vi "Main_GEA3.vi"() -> ()   [LabVIEW 2021]
uses:
  Controles/Multiple_Read_ERD.ctl
  Controles/Read_ERD.ctl
  Controles/Write_Multiple_ERD.ctl
  Controles/Write_ERD.ctl
  Controles/Send_Message.ctl
  Controles/ERD_List.ctl
  Controles/Main_Machine_State.ctl
  Controles/ERD_Data_Boundled.ctl
  Controles/Command(ERD Loop Control).ctl
panel:
  in  "Pause(ms)":u32=100
  out "Rate":u32=100
  in  "Tab Control":enum32{"GEA3", "JSON", "Send Msg", "ERD List"}(tab)
  in  "Write ERD":T1 {"ERD" format="%x"}
  in  "Read ERD":i64[](array[numeric]) format="%x"
  in  "Read":bool
  in  "Write":bool caption="Read"
  in  "dst":i64=192 format="%x"
  out "Multiple_Result":T3 {"ERD Number" format="%x"}
  out "Version":T5
  in  "Json File Path":path
  out "Json":T4[](array[typedef]) {"ERD Number" format="%x"}
  in  "Send":bool caption="Read"
  in  "Send Message":T6={"dst"=192, "Command"=221, "Message"=""} {"Command" format="%x"; "dst" format="%x"}
  out "Message":string
  in  "ERD Default List":T7=[{"Boolean"=TRUE, "ERD Number"=2, "ERD Nanme"="Erd_UnitSerialNumber"}] {"ERD Number" format="%x"}
  in  "ERD's List Ticket Testing":T7=[{"Boolean"=TRUE, "ERD Number"=61497, "ERD Nanme"="Erd_UI_MachineStateEnter"}, {"Boolean"=TRUE, "ERD Number"=61498, "ERD Nanme"="Erd_UI_MachineStateExit"}, {"Boolean"=TRUE, "ERD Number"=61499, "ERD Nanme"="Erd_UI_CycleSelection"}] {"ERD Number" format="%x"}
  in  "Stop Button":bool
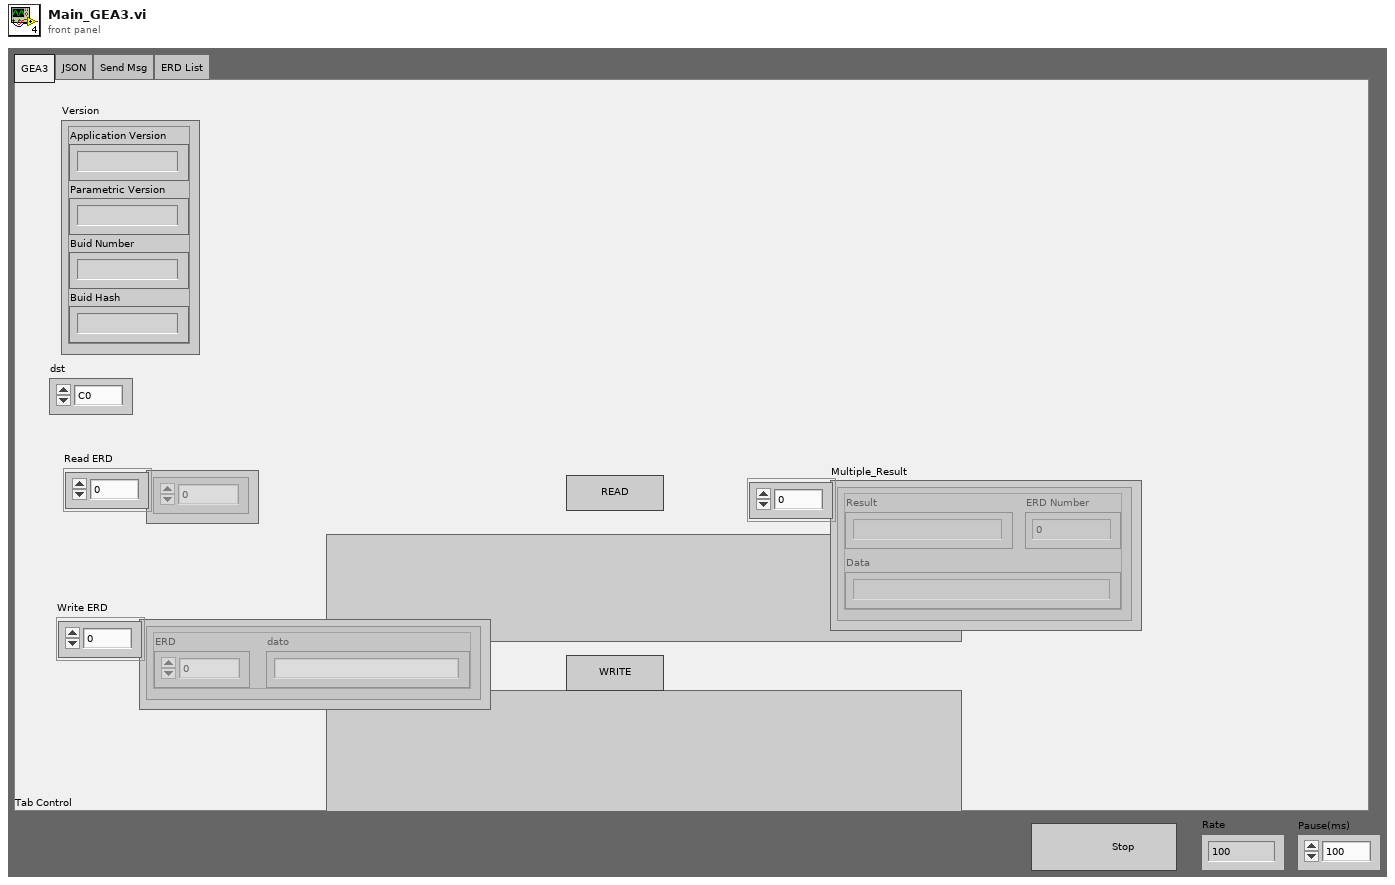
[diagram p1: front panel]
types:
  T1 = typedef "Write_Multiple_ERD.ctl" = T2[]
  T2 = typedef "Write_ERD.ctl" = cluster{"ERD":i64, "dato":string}
  T3 = typedef "Multiple_Read_ERD.ctl" = T4[]
  T4 = typedef "Read_ERD.ctl" = cluster{"Result":string, "ERD Number":i64, "Data":string}
  T5 = cluster{"Application Version":string, "Parametric Version":string, "Buid Number":string, "Buid Hash":string}
  T6 = typedef "Send_Message.ctl" = cluster{"dst":i64, "Command":i64, "Message":string}
  T7 = typedef "ERD_List.ctl" = cluster{"Boolean":bool, "ERD Number":i32, "ERD Nanme":string}[]
  T8 = typedef "ERD_Data_Boundled.ctl" = cluster{"Version":cluster{"Application Version":string, "Parametric Version":string, "Buid Number":string, "Buid Hash":string}}
  T9 = typedef "Main_Machine_State.ctl" = enum16{"Init", "Get Version", "Build ERD Read List", "Update UI", "Read ERDs", "Log Data", "Pause", "Shutdown"}
  T10 = typedef "Command(ERD Loop Control).ctl" = enum16{"Initialize", "Shutdown"}
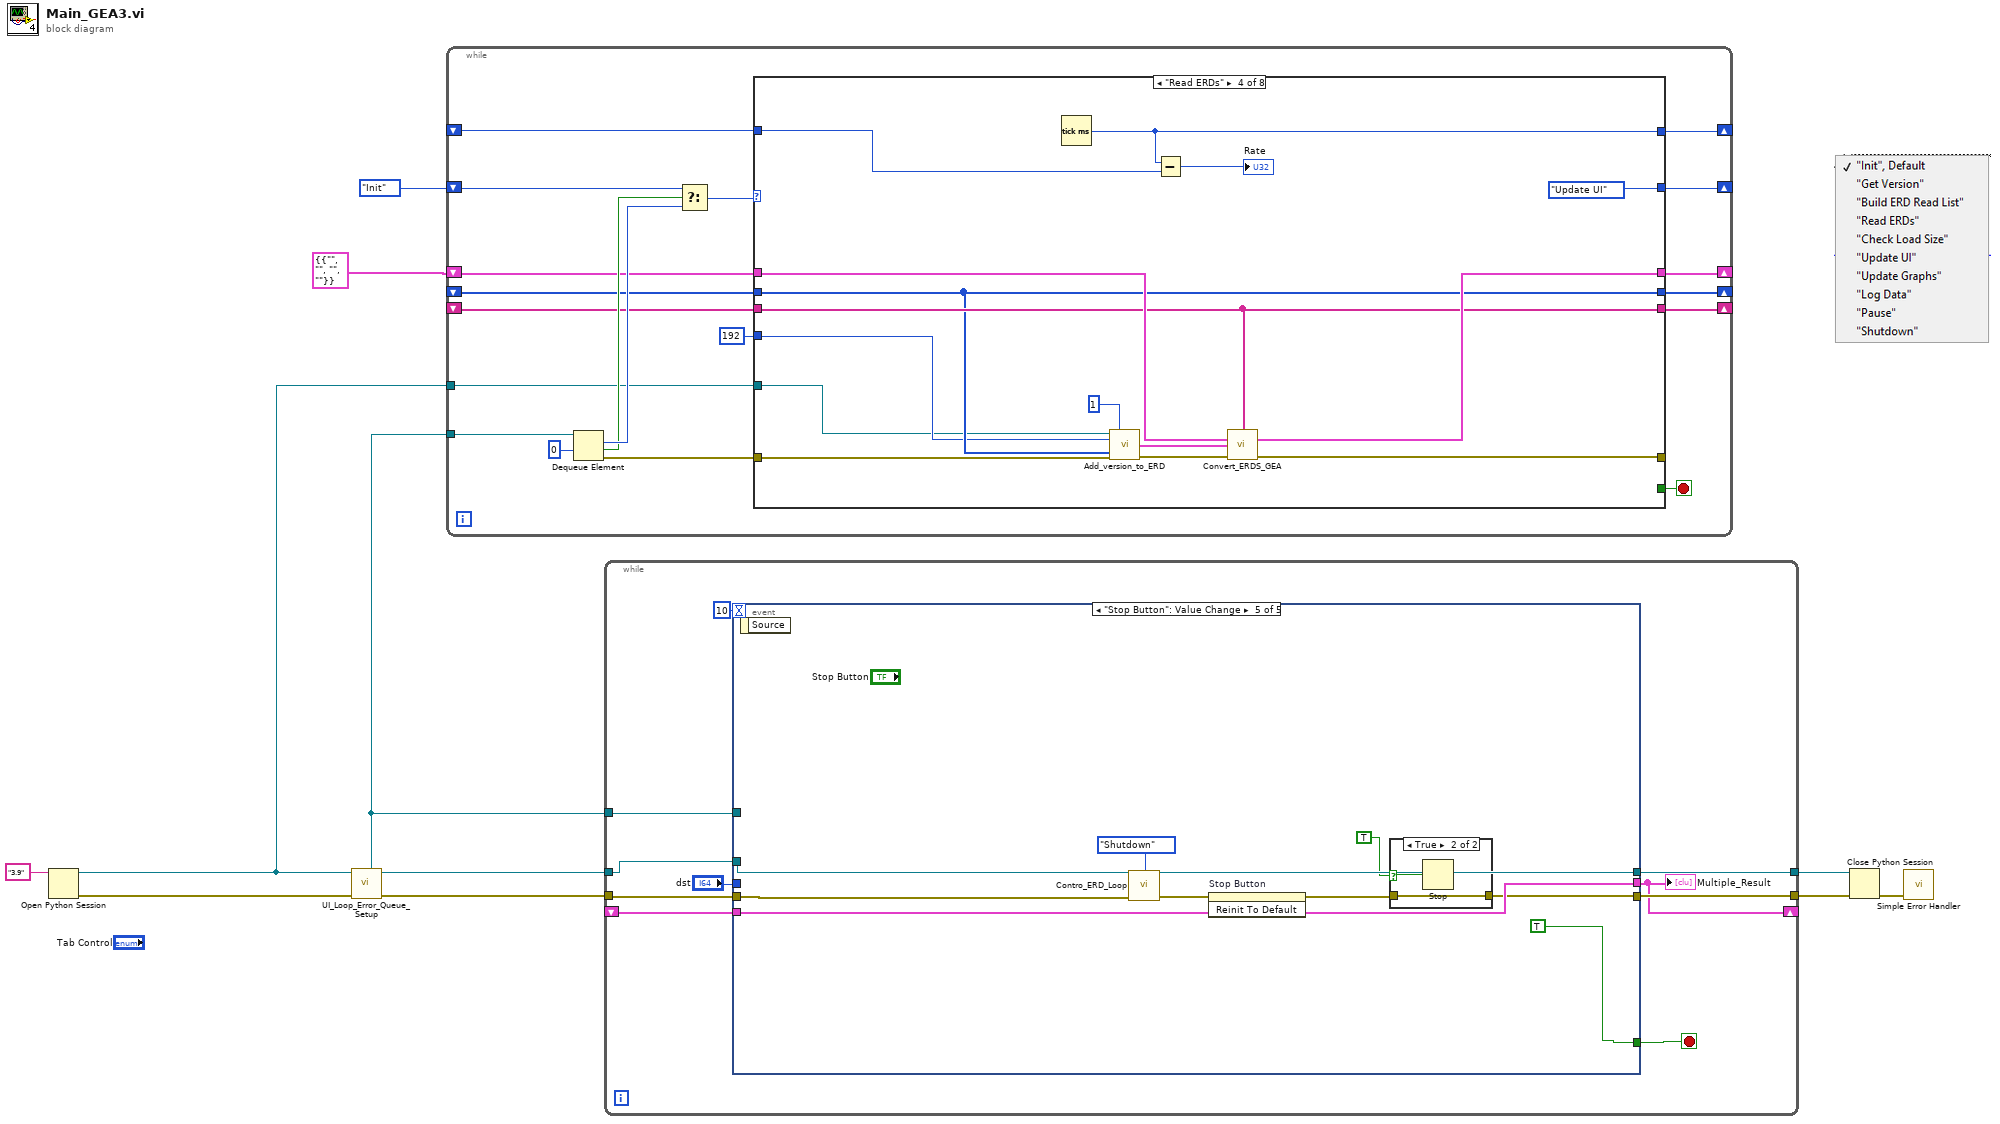
[diagram p0: block diagram]
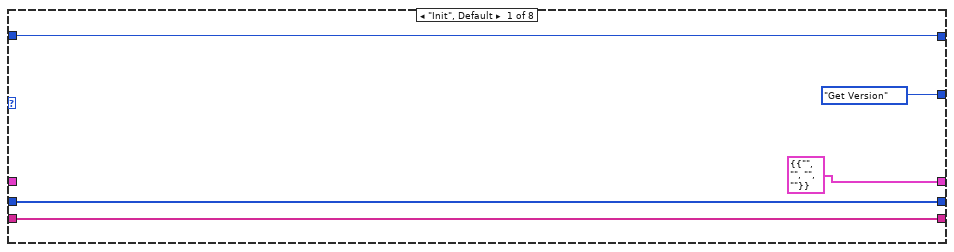
[diagram p2: hidden frame]
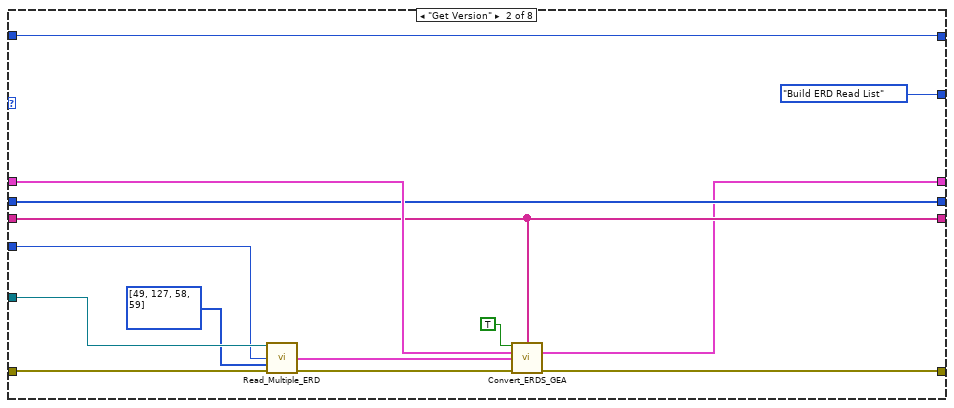
[diagram p3: hidden frame]
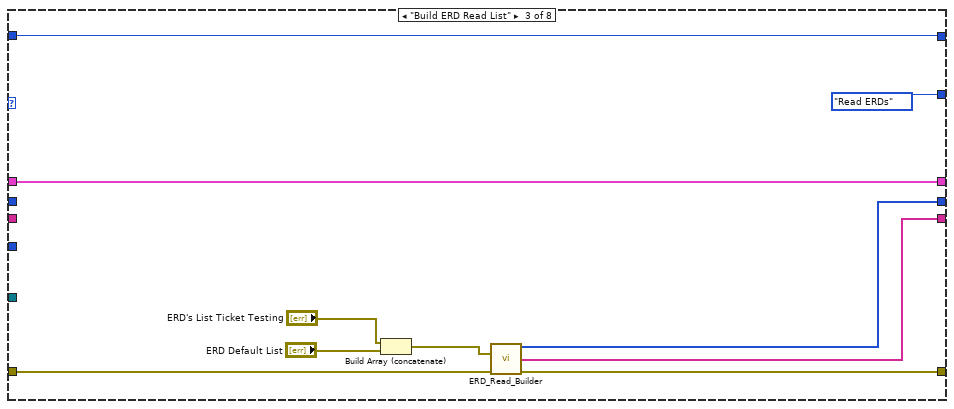
[diagram p4: hidden frame]
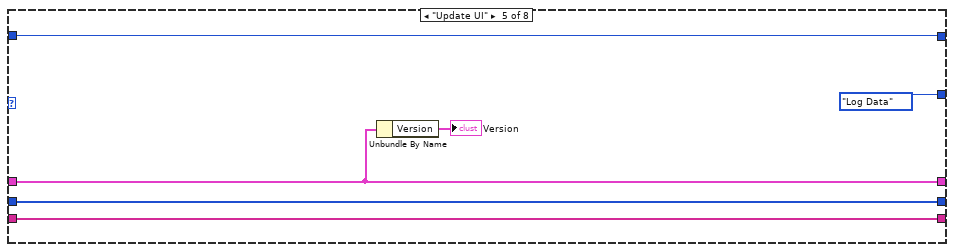
[diagram p5: hidden frame]
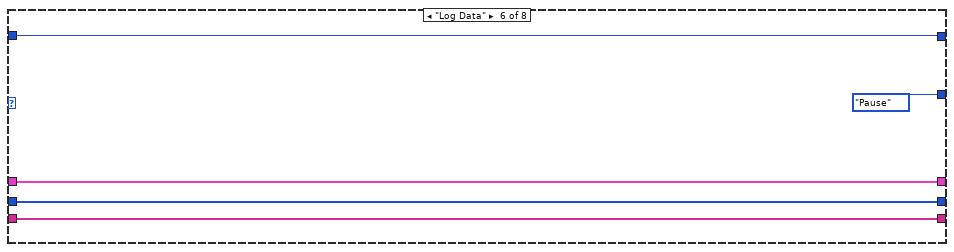
[diagram p6: hidden frame]
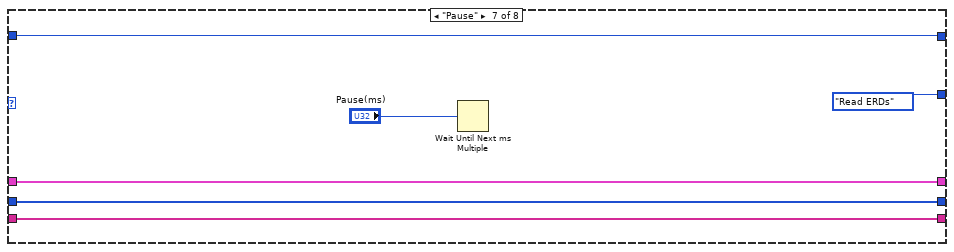
[diagram p7: hidden frame]
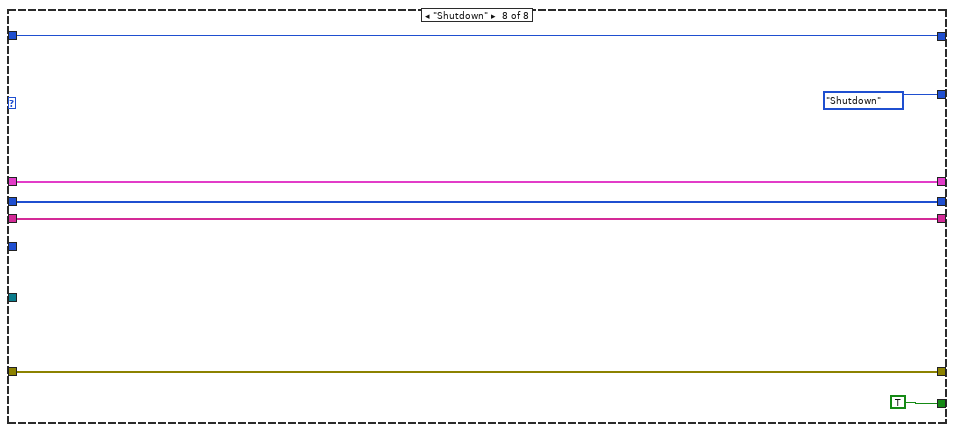
[diagram p8: hidden frame]
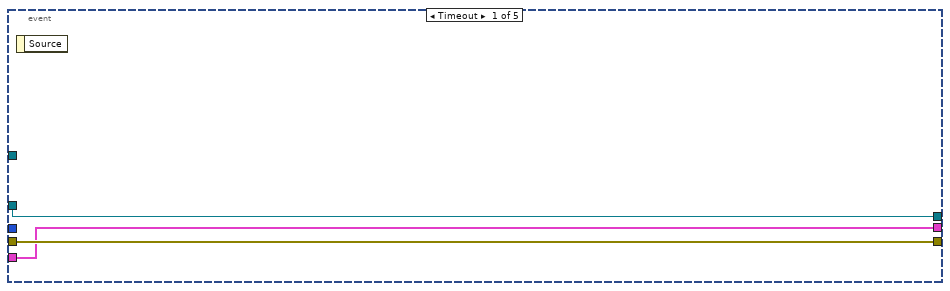
[diagram p9: hidden frame]
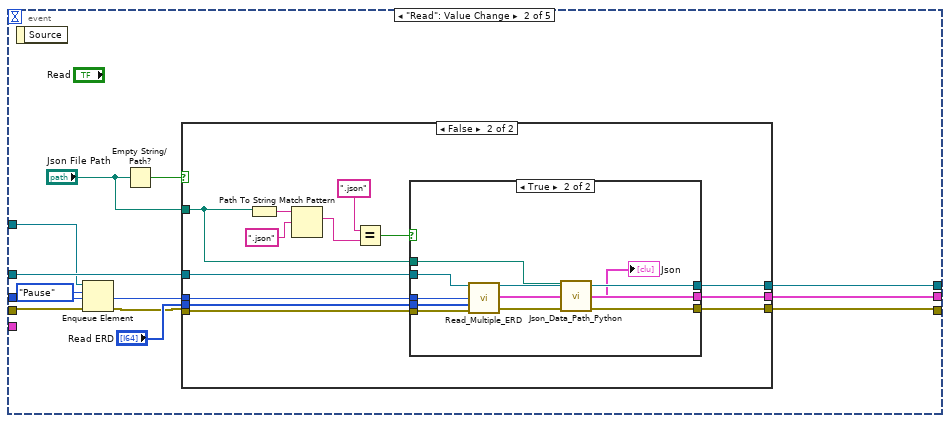
[diagram p10: hidden frame]
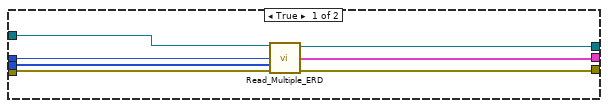
[diagram p11: hidden frame]
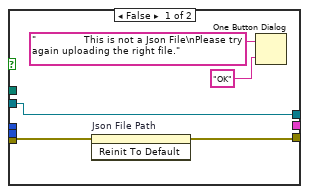
[diagram p12: hidden frame]
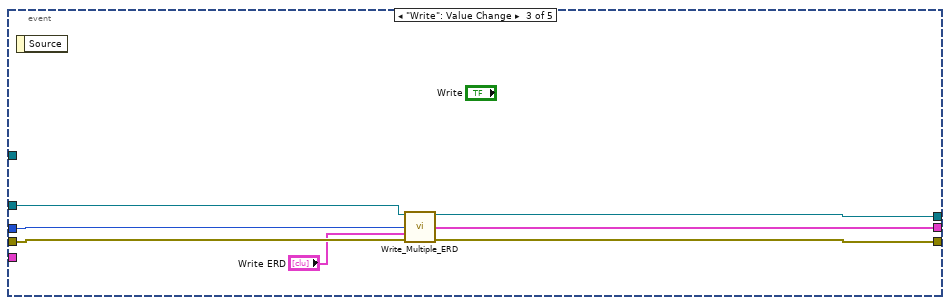
[diagram p13: hidden frame]
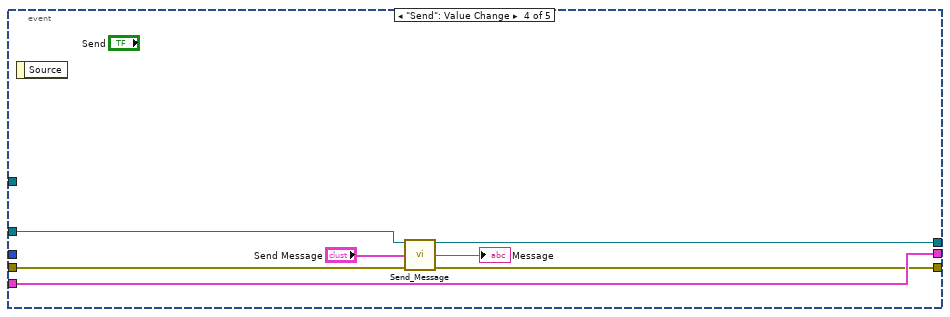
[diagram p14: hidden frame]
diagram:
  n1 = Open Python Session(python version="3.9" ("Python version")) -> (session out=w5:refnum<k35>, error out=w4:errorcluster)  [unwired: 2 in]
  n2 = call "UI_Loop_Error_Queue_Setup.vi"("error in"=w4) -> ("error out"=w6:errorcluster, "queue out"=w3:refnum<queue>)  [unwired: 9 in]
  n3 = while {
    shift-right: [w20] -> _
    shift-left: Main_Machine_State."Init" -> [w27]
    tunnel: w3 -> [w28]
    shift-right: [w23] -> _
    shift-left: _ -> [w22]
    shift-right: [w15] -> _
    shift-left: T8 {"Version"={"Application Version"="", "Parametric Version"="", "Buid Number"="", "Buid Hash"=""}} ("ERD_Data_Bound") -> [w19]
    shift-right: [w17] -> _
    shift-left: _ -> [w14]
    shift-right: [w16] -> _
    shift-left: _ -> [w13]
    tunnel: w5 -> [w12]
    stop <- w21 stop-if-true
    n4 = Dequeue Element(queue=w28, timeout in ms (-1)=0) -> (element=w26:T9, timed out?=w25:bool, error out=w18:errorcluster)  [unwired: 1 in, 1 out]
    n5 = Select(t=w27, s=w25, f=w26) -> (s? t:f=w24:T9)
    n6 = case shown="\"Read ERDs\"" w24 {
      tunnel: [w34 w35 w58 w73 w74 w84 w90 w97] -> w23
      tunnel: w22 -> [w34 w35 w58 w72 w74 w84 w90 w97]
      tunnel: [_ _ _ _ _ _ _ TRUE] -> w21
      tunnel: [Main_Machine_State."Get Version" Main_Machine_State."Build ERD Read List" Main_Machine_State."Read ERDs" Main_Machine_State."Update UI" Main_Machine_State."Log Data" Main_Machine_State."Pause" Main_Machine_State."Read ERDs" Main_Machine_State."Shutdown"] -> w20
      tunnel: w19 -> [_ w43 w49 w69 w78 w82 w87 w91]
      tunnel: w18 -> [_ w47 w54 w65 _ _ _ w94]
      tunnel: [_ w38 w53 w66 _ _ _ w94] -> _
      tunnel: [w32 w41 w51 w64 w77 w81 w86 w92] -> w17
      tunnel: [w31 w40 w50 w67 w76 w80 w85 w93] -> w16
      tunnel: [T8 {"Version"={"Application Version"="", "Parametric Version"="", "Buid Number"="", "Buid Hash"=""}} ("ERD_Data_Bound") w39 w49 w68 w78 w82 w87 w91] -> w15
      tunnel: w14 -> [w32 w41 _ w64 w77 w81 w86 w92]
      tunnel: w13 -> [w31 w40 _ w67 w76 w80 w85 w93]
      tunnel: w12 -> [_ w46 _ w62 _ _ _ _]
      tunnel: i64 192 ("dst") -> [_ w36 _ w63 _ _ _ _]
      frame "Init", Default {
      }
      frame "Get Version" {
        n7 = call "Read_Multiple_ERD.vi"("session in"=w46, "dst"=w36, "Read ERD"=i64[] [49, 127, 58, 59], "error out"=w47) -> ("Multiple Read"=w42:T3, "error IO"=w37:errorcluster)  [unwired: 9 in, 1 out]
        n8 = call "Convert_ERDS_GEA.vi"("New Header?"=TRUE, "ERD Name"=w40, "ERD_Data_Bound"=w43, "Multiple Read"=w42, "error IO"=w37) -> ("All_ERD_Data_Bundled_Brass"=w39:T8, "error out"=w38:errorcluster)  [unwired: 9 in]
      }
      frame "Build ERD Read List" {
        n9 = Build Array (concatenate)("ERD's List Ticket Testing", "ERD Default List") -> (w52:T7)
        n10 = call "ERD_Read_Builder.vi"("ERD Read List All"=w52, "error in"=w54) -> ("Read ERD List"=w51:i32[], "ERD Name"=w50:string[], "error out"=w53:errorcluster)  [unwired: 11 in]
      }
      frame "Read ERDs" {
        n11 = Tick Count (ms)() -> (millisecond timer value=w73:u32)
        n12 = call "Add_version_to_ERD.vi"("session in"=w62, "# of Iterations"=1, "dst"=w63, "Read ERD"=w64, "error in"=w65) -> ("ERD_Data_Out"=w60:T4[], "error out"=w61:errorcluster)  [unwired: 9 in]
        n13 = Subtract(x=w73, y=w72) -> (x-y=→"Rate":u32)
        n14 = call "Convert_ERDS_GEA.vi"("ERD Name"=w67, "ERD_Data_Bound"=w69, "Multiple Read"=w60, "error IO"=w61) -> ("All_ERD_Data_Bundled_Brass"=w68:T8, "error out"=w66:errorcluster)  [unwired: 10 in]
      }
      frame "Update UI" {
        n15 = Unbundle By Name(w78) -> ("Version"=→"Version":T5)
      }
      frame "Log Data" {
      }
      frame "Pause" {
        n16 = Wait Until Next ms Multiple(millisecond multiple="Pause(ms)") -> ()  [unwired: 1 out]
      }
      frame "Shutdown" {
      }
    }
  }
  n17 = while {
    tunnel: w5 -> [w106]
    tunnel: w6 -> [w105]
    tunnel: [w103] -> w9
    tunnel: [w102] -> w8
    shift-right: [w100] -> _
    shift-left: _ -> [w101]
    tunnel: w3 -> [w98]
    stop <- w107 stop-if-true
    n18 = event shown="[4] \"Stop Button\": Value Change" {
      selector: _ -> [_ _ _ _ _]
      dyn-events: _ -> [_ _ _ _ _]
      timeout: 10 -> [_ _ _ _ _]
      tunnel: [_ _ _ _ TRUE] -> w107
      tunnel: w106 -> [w110 w121 w161 w168 w179]
      tunnel: w105 -> [w109 w114 w163 w167 w177]
      tunnel: "dst" -> [_ w120 w162 _ _]
      tunnel: [w110 w122 w159 w170 w179] -> w103
      tunnel: [w109 w117 w164 w169 w174] -> w102
      tunnel: [w108 w118 w158 w171 w178] -> w100
      tunnel: w101 -> [w108 _ _ w171 w178]
      tunnel: w98 -> [_ w112 _ _ _]
      event Timeout {
        n19 = event-data() -> ()  [unwired: 1 in, 1 out]
      }
      event "Read": Value Change {
        n20 = event-data() -> ()  [unwired: 1 in, 1 out]
        n21 = Enqueue Element(queue=w112, element=Main_Machine_State."Pause", error in (no error)=w114) -> (error out=w113:errorcluster)  [unwired: 1 in, 2 out]
        n22 = Empty String/Path?(string/path="Json File Path") -> (empty?=w116:bool)
        n23 = case shown="False" w116 {
          tunnel: w113 -> [w128 w142]
          tunnel: [w126 w141] -> w122
          tunnel: w121 -> [w129 w140]
          tunnel: w120 -> [w124 w139]
          tunnel: "Read ERD" -> [w123 w138]
          tunnel: [w125 w137] -> w118
          tunnel: [w127 w136] -> w117
          tunnel: "Json File Path" -> [_ w132]
          frame True {
            n24 = call "Read_Multiple_ERD.vi"("session in"=w129, "dst"=w124, "Read ERD"=w123, "error out"=w128) -> ("session out"=w126:refnum<k35>, "Multiple Read"=w125:T3, "error IO"=w127:errorcluster)  [unwired: 9 in]
          }
          frame False {
            n25 = Path To String(path=w132) -> (string=w134:string)
            n26 = Match Pattern(string=w134, regular expression=".json") -> (match substring=w130:string)  [unwired: 1 in, 3 out]
            n27 = Equal?(x=".json", y=w130) -> (x = y?=w133:bool)
            n28 = case shown="True" w133 {
              tunnel: w142 -> [w144 w157]
              tunnel: [w147 w156] -> w141
              tunnel: w140 -> [w147 w155]
              tunnel: w139 -> [_ w154]
              tunnel: w138 -> [_ w153]
              tunnel: [_ w152] -> w137
              tunnel: [w143 w150] -> w136
              tunnel: w132 -> [_ w148]
              frame False {
                n29 = invoke on="Json File Path" class="Path" method="Reinit To Default"(error in=w144) -> (error out=w143:errorcluster)  [unwired: 2 in, 2 out]
                n30 = One Button Dialog(message="                This is not a Json File\nPlease try again uploading the right file.", button name ("OK")="OK") -> ()  [unwired: 1 out]
              }
              frame True {
                n31 = call "Read_Multiple_ERD.vi"("session in"=w155, "dst"=w154, "Read ERD"=w153, "error out"=w157) -> ("session out"=w156:refnum<k35>, "Multiple Read"=w152:T3, "error IO"=w151:errorcluster)  [unwired: 9 in]
                n32 = call "Json_Data_Path_Python.vi"("Json File Path"=w148, "Multiple Read"=w152, "error in"=w151) -> ("Multiple Read 2"=→"Json":T4[], "error out"=w150:errorcluster)  [unwired: 11 in]
              }
            }
          }
        }
      }
      event "Write": Value Change {
        n33 = event-data() -> ()  [unwired: 1 in, 1 out]
        n34 = call "Write_Multiple_ERD.vi"("session in"=w161, "dst"=w162, "Write ERD"="Write ERD", "error out"=w163) -> ("session out"=w159:refnum<k35>, "Multiple Read"=w158:T3, "error IO"=w164:errorcluster)  [unwired: 9 in]
      }
      event "Send": Value Change {
        n35 = event-data() -> ()  [unwired: 1 in, 1 out]
        n36 = call "Send_Message.vi"("session in"=w168, "Send Message"="Send Message", "error in (no error)"=w167) -> ("session out"=w170:refnum<k35>, "Message"=→"Message":string, "error out"=w169:errorcluster)  [unwired: 10 in]
      }
      event "Stop Button": Value Change {
        n37 = event-data() -> ()  [unwired: 1 in, 1 out]
        n38 = call "Contro_ERD_Loop.vi"("Error In"=w177, "Command (ERD Loop Control)"=Command(ERD_Loop_Control)."Shutdown") -> ("Error Out"=w173:errorcluster)  [unwired: 13 in]
        n39 = invoke on="Stop Button" class="Bool" method="Reinit To Default"(error in=w173) -> (error out=w172:errorcluster)  [unwired: 2 in, 2 out]
        n40 = case shown="True" TRUE {
          selector: TRUE -> [_ w182]
          tunnel: w172 -> [w181 w183]
          tunnel: [w181 w183] -> w174
          frame False {
          }
          frame True {
            n41 = Stop(stop? (T)=w182) -> ()
          }
        }
      }
    }
    "Multiple_Result" <- w100
  }
  n42 = Close Python Session(session in=w9, error in=w8) -> (11:w7:errorcluster)
  n43 = call <vilib>:"Simple Error Handler.vi"("error in (no error)"=w7) -> ()  [unwired: 4 in, 5 out]
